vi "Write Multiple.vi"(8 "error in (no error)":errorcluster, 9 "Values":variant[](array[variant]), 10 "Symbol Names":string[](array[string]), 11 "TwinCAT ADS in":refnum<class "TwinCAT ADS.lvclass">) -> (0 "error out":errorcluster, 3 "TwinCAT ADS out":refnum<class "TwinCAT ADS.lvclass">)   [LabVIEW 2018, in "TwinCAT ADS.lvclass"]
uses:
  TwinCAT ADS.lvclass
  TwinCAT ADS.lvclass/TwinCAT ADS.ctl
  TwinCAT.Ads
  Get From Symbol Map.vi
  Get From Symbol Map Daemon.vi
  Get Symbol Map.vi
  Format String.vi
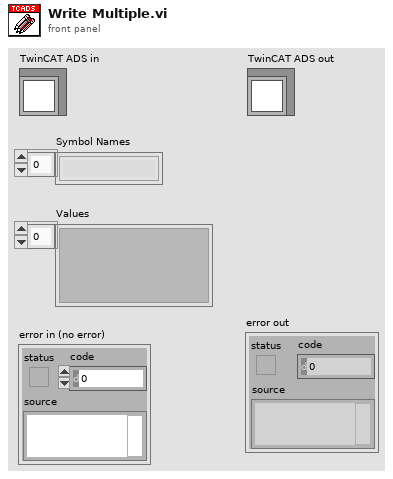
[diagram p1: front panel]
types:
  T1 = enum16{"big-endian, network order", "native, host order", "little-endian"}
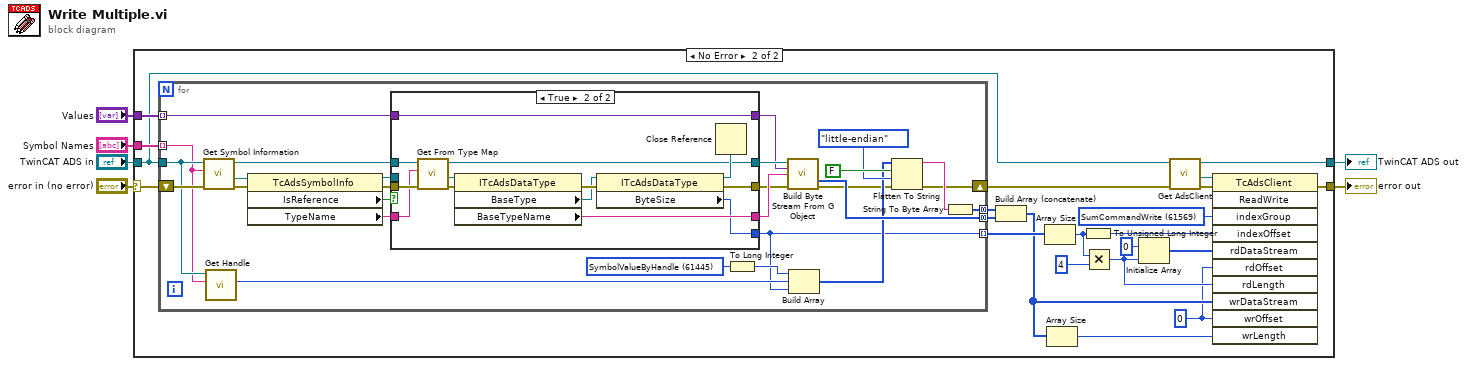
[diagram p0: block diagram]
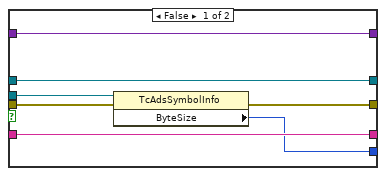
[diagram p3: hidden frame]
diagram:
  n1 = case shown="No Error" "error in (no error)" {
    selector: "error in (no error)" -> [w7 w9]
    tunnel: "Values" -> [_ w30]
    tunnel: "Symbol Names" -> [_ w29]
    tunnel: "TwinCAT ADS in" -> [w8 w10]
    tunnel: [w7 w12] -> w3
    tunnel: [w8 w11] -> w2
    frame Error {
    }
    frame No Error {
      w13 = 0 ("wrOffset")
      w23 = u32 61569 items=["PlcRWIB"=16384, "PlcRWOB"=16400, "PlcRWMB"=16416, "PlcRWRB"=16432, "PlcRWDB"=16448, "SymbolTable"=61440, "SymbolName"=61441, "SymbolValue"=61442, "SymbolHandleByName"=61443, "SymbolValueByName"=61444, "SymbolValueByHandle"=61445, "SymbolReleaseHandle"=61446, "SymbolInfoByName"=61447, "SymbolVersion"=61448, "SymbolInfoByNameEx"=61449, "SymbolDownload"=61450, "SymbolUpload"=61451, "SymbolUploadInfo"=61452, "SymbolNote"=61456, "IOImageRWIB"=61472, "IOImageRWIX"=61473, "IOImageRWOB"=61488, "IOImageRWOX"=61489, "IOImageClearI"=61504, "IOImageClearO"=61520, "SumCommandRead"=61568, "SumCommandWrite"=61569, "SumCommandReadWrite"=61570, "SumCommandReadEx"=61571, "SumCommandReadEx2"=61572, "SumCommandAddDevNote"=61573, "SumCommandDelDevNote"=61574, "DeviceData"=61696] ("SumCommandRead")
      n2 = for {
        tunnel: w29 -> [w37] mode=indexing
        tunnel: [w38] -> w22 mode=indexing
        shift-right: [w35] -> w24
        shift-left: w9 -> [w56]
        tunnel: [w50] -> w28 mode=concatenating
        tunnel: w30 -> [w41] mode=indexing
        tunnel: [w49] -> w27 mode=concatenating
        tunnel: w10 -> [w54]
        w48 = u32 61445 items=["PlcRWIB"=16384, "PlcRWOB"=16400, "PlcRWMB"=16416, "PlcRWRB"=16432, "PlcRWDB"=16448, "SymbolTable"=61440, "SymbolName"=61441, "SymbolValue"=61442, "SymbolHandleByName"=61443, "SymbolValueByName"=61444, "SymbolValueByHandle"=61445, "SymbolReleaseHandle"=61446, "SymbolInfoByName"=61447, "SymbolVersion"=61448, "SymbolInfoByNameEx"=61449, "SymbolDownload"=61450, "SymbolUpload"=61451, "SymbolUploadInfo"=61452, "SymbolNote"=61456, "IOImageRWIB"=61472, "IOImageRWIX"=61473, "IOImageRWOB"=61488, "IOImageRWOX"=61489, "IOImageClearI"=61504, "IOImageClearO"=61520, "SumCommandRead"=61568, "SumCommandWrite"=61569, "SumCommandReadWrite"=61570, "SumCommandReadEx"=61571, "SumCommandReadEx2"=61572, "SumCommandAddDevNote"=61573, "SumCommandDelDevNote"=61574, "DeviceData"=61696] ("SumCommandRead")
        n3 = call "Get Symbol Information.vi"("error in (no error)"=w56, "Symbol Name"=w37, "TwinCAT ADS in"=w54) -> ("error out"=w36:errorcluster, ".NET Symbol Information"=w55:refnum<k24>, "TwinCAT ADS out"=w45:refnum<class "TwinCAT ADS.lvclass">)  [unwired: 6 in]
        n4 = call "Get Handle.vi"("Symbol Name"=w37, "TwinCAT ADS in"=w54) -> ("Handle"=w57:i32)  [unwired: 7 in, 2 out]
        n5 = property class="TcAdsSymbolInfo"(reference=w55, error in=w36) -> (reference out=w31:refnum<k24>, error out=w32:errorcluster, "IsReference"=w44:bool, "TypeName"=w43:string)
        n6 = case shown="True" w44 {
          tunnel: w32 -> [w61 w77]
          tunnel: w43 -> [w62 w74]
          tunnel: [w62 w68] -> w39
          tunnel: [w58 w66] -> w38
          tunnel: [w60 w70] -> w33
          tunnel: w45 -> [w64 w69]
          tunnel: [w64 w67] -> w42
          tunnel: w41 -> [w63 w65]
          tunnel: [w63 w65] -> w40
          tunnel: w31 -> [w59 _]
          frame False {
            n7 = property class="TcAdsSymbolInfo"(reference=w59, error in=w61) -> (error out=w60:errorcluster, "ByteSize"=w58:i32)  [unwired: 1 out]
          }
          frame True {
            n8 = call "Get From Type Map.vi"("error in (no error)"=w77, "Type Name"=w74, "TwinCAT ADS in"=w69) -> ("error out"=w76:errorcluster, ".NET AdsDataType"=w75:refnum<k24>, "TwinCAT ADS out"=w67:refnum<class "TwinCAT ADS.lvclass">)  [unwired: 6 in]
            n9 = property class="ITcAdsDataType"(reference=w75, error in=w76) -> (error out=w73:errorcluster, "BaseType"=w72:refnum<k24>, "BaseTypeName"=w68:string)  [unwired: 1 out]
            n10 = property class="ITcAdsDataType"(reference=w72, error in=w73) -> (reference out=w71:refnum<k24>, error out=w70:errorcluster, "ByteSize"=w66:i32)
            n11 = Close Reference(reference=w71) -> ()  [unwired: 1 in, 1 out]
          }
        }
        n12 = To Long Integer(number=w48) -> (32bit integer=w47:i32)
        n13 = call "Build Byte Stream From G Object.vi"("TwinCAT ADS in"=w42, "Value"=w40, "Type Name"=w39, "error in (no error)"=w33) -> ("Byte Stream out"=w49:u8[], "error out"=w34:errorcluster)  [unwired: 9 in, 1 out]
        n14 = Build Array(w47, w57, w38) -> (w46:i32[])
        n15 = Flatten To String(anything=w46, prepend array or string size? (T)=FALSE, byte order (0:big-endian, network order)=T1."little-endian" ("Byte Order (little-endian)"), error in (no error)=w34) -> (data string=w53:string, error out=w35:errorcluster)  [unwired: 1 out]
        n16 = String To Byte Array(string=w53) -> (unsigned byte array=w50:u8[])
      }
      n17 = Build Array (concatenate)(w28, w27) -> (w15:u8[])
      n18 = Array Size(array=w22) -> (size(s)=w17:i32)
      n19 = Array Size(array=w15) -> (size(s)=w14:i32)
      n20 = To Unsigned Long Integer(number=w17) -> (unsigned 32bit integer=w21:u32)
      n21 = Multiply(x=w17, y=4 ("length")) -> (x*y=w16:i32)
      n22 = Initialize Array(u8 0, w16) -> (w19:u8[])
      n23 = call "Get AdsClient.vi"("error in (no error)"=w24, "TwinCAT ADS in"=w10) -> ("error out"=w26:errorcluster, ".NET TcAdsClient"=w25:refnum<k24>, "TwinCAT ADS out"=w11:refnum<class "TwinCAT ADS.lvclass">)  [unwired: 7 in]
      n24 = invoke class="TcAdsClient" method="ReadWrite"(reference=w25, error in=w26, "indexGroup"=w23, "indexOffset"=w21, "rdDataStream"=w19, "rdOffset"=w13, "rdLength"=w16, "wrDataStream"=w15, "wrOffset"=w13, "wrLength"=w14) -> (error out=w12:errorcluster)  [unwired: 1 in, 10 out]
    }
  }
  "error out" <- w3
  "TwinCAT ADS out" <- w2
